vi "Set Mode.vi"(0 "TCS.lvclass in":refnum<class "TCS.lvclass">, 1 "On&G 0":T1, 2 "On&G 1":T1, 3 "On&G 2":T1, 4 "On&G 3":T1, 5 "error in (no error)":errorcluster) -> (14 "TCS.lvclass out":refnum<class "TCS.lvclass">, 19 "error out":errorcluster)   [LabVIEW 2016, in "TCS.lvclass"]
uses:
  Lib.llb/TCS.lvclass
  Lib.llb/CS.lvclass
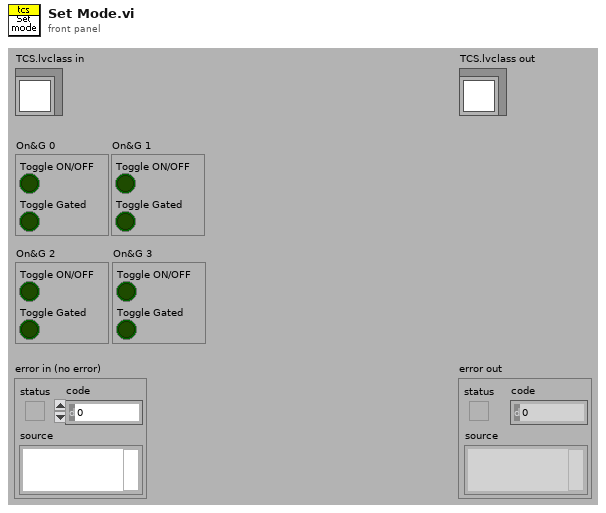
[diagram p1: front panel]
types:
  T1 = cluster{"Toggle ON/OFF":bool, "Toggle Gated":bool}
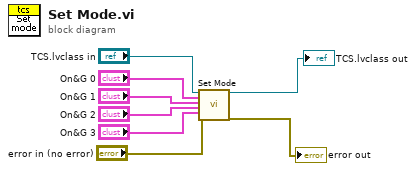
[diagram p0: block diagram]
diagram:
  n1 = call-parent "Set Mode.vi"("CS.lvclass in"="TCS.lvclass in", "On&G 0"="On&G 0", "On&G 1"="On&G 1", "On&G 2"="On&G 2", "On&G 3"="On&G 3", "error in (no error)"="error in (no error)") -> ("CS.lvclass out"=→"TCS.lvclass out":refnum<class "TCS.lvclass">, "error out"=→"error out":errorcluster)  [unwired: 12 in]
